vi "Parse DB - 1553 - Get BM Config.vi"(0 "channel config handle":u32, 11 "error in (no error)":errorcluster) -> (4 "channel config handle out":u32, 6 "Bus_Monitor":T1, 8 "Address Set Inverted":bool, 15 "error out":errorcluster)   [LabVIEW 2013, in "AIT 1553 Custom Device.lvlib"]
uses:
  AIT 1553 Custom Device.lvlib
  Controls/1553_Bus_Monitor.ctl
  Controls/1553_BM_Message.ctl
  Controls/1553 Param.ctl
  Controls/1553_Bus_Controller.ctl
  Controls/1553_BC_Message.ctl
  Controls/1553_Acyclic_Frame.ctl
  <userlib>/MIL-STD-1553/Owl1553.lvlib
panel:
  out "BM Tx Array":bool[][](array[boolean])
  out "BM Rx Array":bool[][](array[boolean])
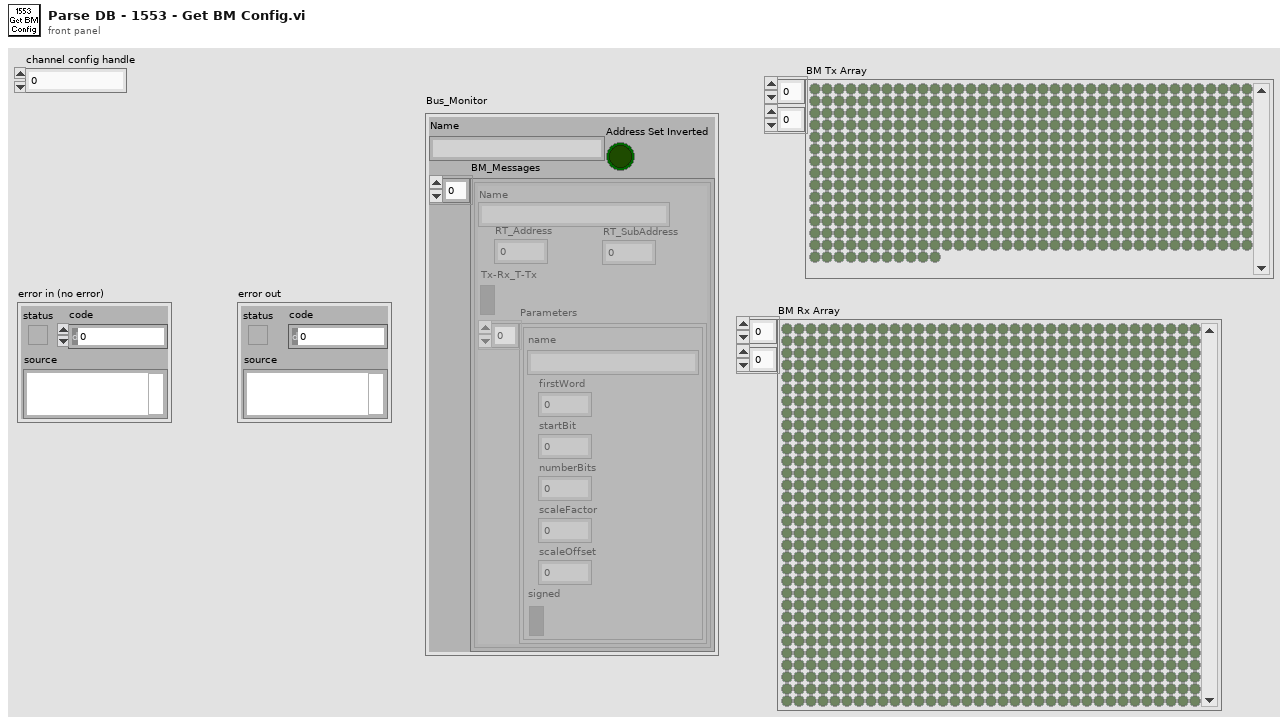
[diagram p1: front panel]
types:
  T1 = typedef "AIT 1553 Custom Device.lvlib/1553_Bus_Monitor.ctl" = cluster{"Name":string, "BM_Messages":T2[], "Address Set Inverted":bool}
  T2 = typedef "AIT 1553 Custom Device.lvlib/1553_BM_Message.ctl" = cluster{"RT_Address":u8, "RT_SubAddress":u8, "Tx-Rx_T-Tx":bool, "Parameters":T3[], "Name":string}
  T3 = typedef "AIT 1553 Custom Device.lvlib/1553 Param.ctl" = cluster{"name":string, "firstWord":i32, "startBit":i32, "numberBits":i32, "scaleFactor":dbl, "scaleOffset":dbl, "signed":bool}
  T4 = typedef "AIT 1553 Custom Device.lvlib/1553_Bus_Controller.ctl" = cluster{"BC_Messages":T5[], "Acyclic_Frames":T6[], "Enabled":bool}
  T5 = typedef "AIT 1553 Custom Device.lvlib/1553_BC_Message.ctl" = cluster{"Name":string, "Tx-Rx_T-Tx":bool, "RT_Address":u8, "RT_SA_Address":u8, "Parameters":T3[], "Transfer Enabled":bool, "Message Buffer ID":u16, "Default_Message_Buffer_Data":u16[], "Word_Count":u8}
  T6 = typedef "AIT 1553 Custom Device.lvlib/1553_Acyclic_Frame.ctl" = cluster{"Frame_Index":u8, "Initiate_Xfer":bool}
  T7 = enum16{"OWL1553_RECEIVE_TRANSFER", "OWL1553_TRANSMIT_TRANSFER"}
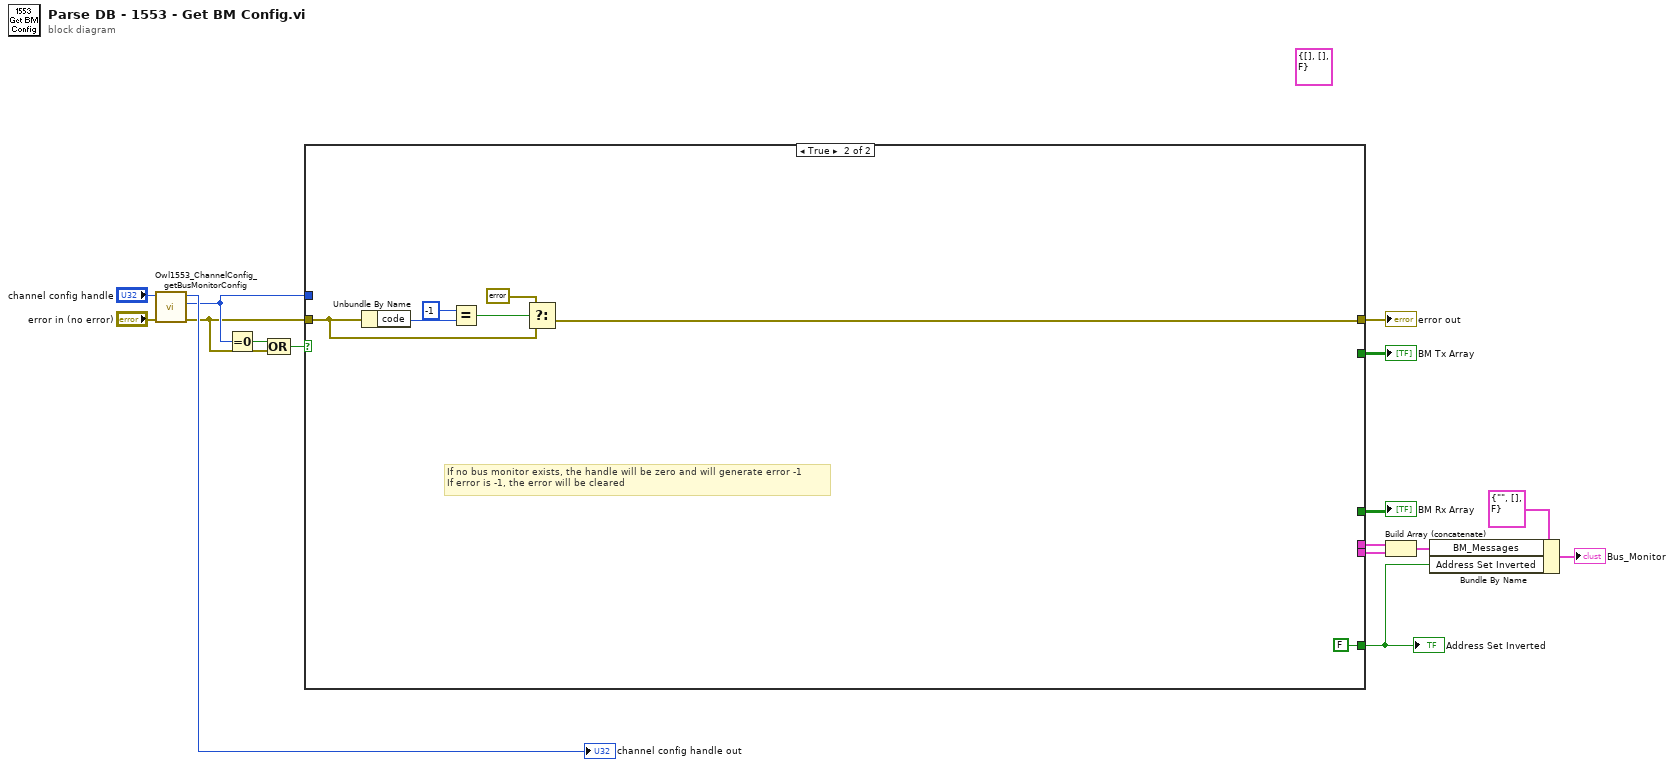
[diagram p0: block diagram]
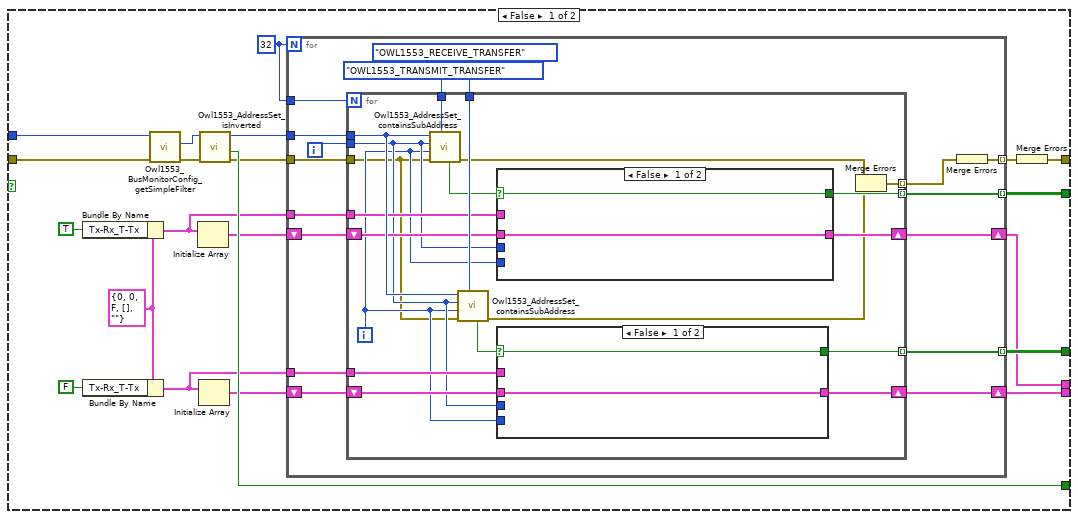
[diagram p2: hidden frame]
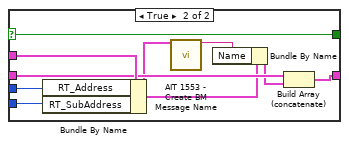
[diagram p3: hidden frame]
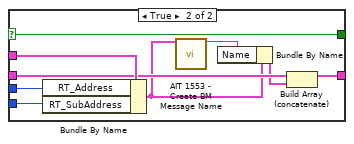
[diagram p4: hidden frame]
diagram:
  (unwired) T4 {"BC_Messages"=[], "Acyclic_Frames"=[], "Enabled"=FALSE} ("Bus_Controller")
  n1 = call <userlib>:"Owl1553_ChannelConfig_getBusMonitorConfig.vi"("error in (no error)"="error in (no error)", "channel config handle"="channel config handle") -> ("error out"=w2:errorcluster, "bus monitor config handle"=w4:u32, "channel config handle"=→"channel config handle out":u32)  [unwired: 7 in]
  n2 = Equal To 0?(x=w4) -> (x = 0?=w3:bool)
  n3 = Compound Arithmetic op=OR(w3, w2) -> (w1:bool)
  n4 = case shown="True" w1 {
    tunnel: [w36 _] -> w15
    tunnel: [w35 _] -> w14
    tunnel: w2 -> [w34 w97]
    tunnel: w4 -> [w33 _]
    tunnel: [w30 FALSE ("inverted")] -> w10
    tunnel: [w22 _] -> w9
    tunnel: [w21 _] -> w8
    tunnel: [w17 w95] -> w5
    frame False {
      w26 = T2 {"RT_Address"=0, "RT_SubAddress"=0, "Tx-Rx_T-Tx"=FALSE, "Parameters"=[], "Name"=""} ("BM_Message")
      w37 = 32
      n5 = Bundle By Name(cluster=w26, "Tx-Rx_T-Tx"=TRUE ("Tx-Rx (T=Tx)")) -> (w24:T2)
      n6 = Bundle By Name(cluster=w26, "Tx-Rx_T-Tx"=FALSE ("Tx-Rx (T=Tx)")) -> (w23:T2)
      n7 = call <userlib>:"Owl1553_BusMonitorConfig_getSimpleFilter.vi"("error in (no error)"=w34, "config handle"=w33) -> ("error out"=w32:errorcluster, "address set handle"=w20:u32)  [unwired: 7 in, 1 out]
      n8 = Initialize Array(w24) -> (w29:T2[])  [unwired: 1 in]
      n9 = Initialize Array(w23) -> (w25:T2[])  [unwired: 1 in]
      n10 = call <userlib>:"Owl1553_AddressSet_isInverted.vi"("error in (no error)"=w32, "address set handle"=w20) -> ("error out"=w19:errorcluster, "inverted"=w30:bool, "address set handle"=w31:u32)  [unwired: 7 in]
      n11 = for {
        N: w37 -> [_]
        tunnel: w31 -> [w53]
        tunnel: [w52] -> w35 mode=indexing
        tunnel: w37 -> [w50]
        tunnel: [w47] -> w36 mode=indexing
        shift-right: [w44] -> w21
        shift-left: w29 -> [w45]
        shift-right: [w41] -> w22
        shift-left: w25 -> [w43]
        tunnel: w24 -> [w46]
        tunnel: w23 -> [w42]
        tunnel: w19 -> [w40]
        tunnel: [w38] -> w18 mode=indexing
        i -> [w51]
        n12 = for {
          N: w50 -> [_]
          tunnel: w53 -> [w72]
          tunnel: [w66] -> w52 mode=indexing
          tunnel: w51 -> [w59]
          tunnel: T7."OWL1553_TRANSMIT_TRANSFER" ("direction") -> [w70]
          tunnel: T7."OWL1553_RECEIVE_TRANSFER" ("direction") -> [w71]
          tunnel: [w63] -> w47 mode=indexing
          tunnel: w46 -> [w69]
          shift-right: [w65] -> w44
          shift-left: w45 -> [w68]
          shift-right: [w60] -> w41
          shift-left: w43 -> [w62]
          tunnel: w42 -> [w61]
          tunnel: w40 -> [w55]
          tunnel: [w54] -> w39 mode=indexing
          i -> [w58]
          n13 = call <userlib>:"Owl1553_AddressSet_containsSubAddress.vi"("direction"=w70, "error in (no error)"=w55, "sub address"=w58, "remote terminal address"=w59, "address set handle"=w72) -> ("error out"=w57:errorcluster, "contains sub-address"=w67:bool)  [unwired: 4 in, 1 out]
          n14 = call <userlib>:"Owl1553_AddressSet_containsSubAddress.vi"("direction"=w71, "error in (no error)"=w55, "sub address"=w58, "remote terminal address"=w59, "address set handle"=w72) -> ("error out"=w56:errorcluster, "contains sub-address"=w64:bool)  [unwired: 4 in, 1 out]
          n15 = case shown="False" w67 {
            selector: w67 -> [w84 w93]
            tunnel: w69 -> [_ w94]
            tunnel: w68 -> [w85 w92]
            tunnel: [w84 w93] -> w66
            tunnel: [w85 w91] -> w65
            tunnel: w59 -> [_ w90]
            tunnel: w58 -> [_ w89]
            frame False {
            }
            frame True {
              n16 = Bundle By Name(cluster=w94, "RT_Address"=w90, "RT_SubAddress"=w89) -> (w87:T2)
              n17 = call "AIT 1553 - Create BM Message Name.vi"("BM_Message"=w87) -> ("Message Name"=w88:string)  [unwired: 13 in, 1 out]
              n18 = Bundle By Name(cluster=w87, "Name"=w88) -> (w86:T2)
              n19 = Build Array (concatenate)(w92, w86) -> (w91:T2[])
            }
          }
          n20 = case shown="False" w64 {
            selector: w64 -> [w73 w82]
            tunnel: w61 -> [_ w83]
            tunnel: w62 -> [w74 w81]
            tunnel: [w73 w82] -> w63
            tunnel: [w74 w80] -> w60
            tunnel: w59 -> [_ w79]
            tunnel: w58 -> [_ w78]
            frame False {
            }
            frame True {
              n21 = Bundle By Name(cluster=w83, "RT_Address"=w79, "RT_SubAddress"=w78) -> (w76:T2)
              n22 = call "AIT 1553 - Create BM Message Name.vi"("BM_Message"=w76) -> ("Message Name"=w77:string)  [unwired: 13 in, 1 out]
              n23 = Bundle By Name(cluster=w76, "Name"=w77) -> (w75:T2)
              n24 = Build Array (concatenate)(w81, w75) -> (w80:T2[])
            }
          }
          n25 = Merge Errors(w57, w56) -> (w54:errorcluster)
        }
        n26 = Merge Errors(w39) -> (w38:errorcluster)
      }
      n27 = Merge Errors(w18) -> (w17:errorcluster)
    }
    frame True {
      # "If no bus monitor exists, the handle will be zero and will generate error -1\nIf error is -1, the error will be cleared"
      n28 = Unbundle By Name(w97) -> ("code"=w100:i32)
      n29 = Equal?(x=-1, y=w100) -> (x = y?=w98:bool)
      n30 = Select(t=errorcluster {"status"=FALSE, "code"=0, "source"=""} ("error out"), s=w98, f=w97) -> (s? t:f=w95:errorcluster)
    }
  }
  "error out" <- w5
  "BM Tx Array" <- w14
  "BM Rx Array" <- w15
  "Address Set Inverted" <- w10
  n31 = Build Array (concatenate)(w8, w9) -> (w7:T2[])
  n32 = Bundle By Name(cluster=T1 {"Name"="", "BM_Messages"=[], "Address Set Inverted"=FALSE} ("Bus_Monitor"), "BM_Messages"=w7, "Address Set Inverted"=w10) -> (→"Bus_Monitor":T1)
